vi "Communication - TD PID Data (FGV).vi"(7 "Action":T2=enum."Write", 8 "error in (no error)":errorcluster, 11 "TD PID SV":T1) -> (0 "error out":errorcluster, 3 "TD PID SV out":T1)   [LabVIEW 2019]
uses:
  Controls/FGV States.ctl
  Controls/Communication - TD PID.ctl
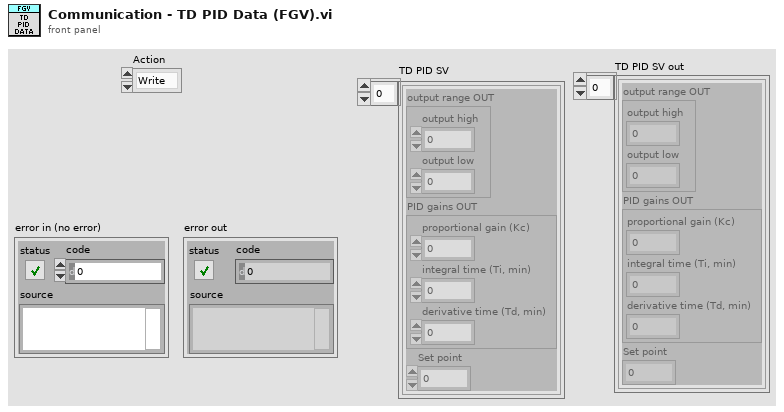
[diagram p1: front panel]
types:
  T1 = typedef "Communication - TD PID.ctl" = cluster{"output range OUT":cluster{"output high":dbl, "output low":dbl}, "PID gains OUT":cluster{"proportional gain (Kc)":dbl, "integral time (Ti, min)":dbl, "derivative time (Td, min)":dbl}, "Set point":dbl}[]
  T2 = typedef "FGV States.ctl" = enum16{"Read", "Write"}
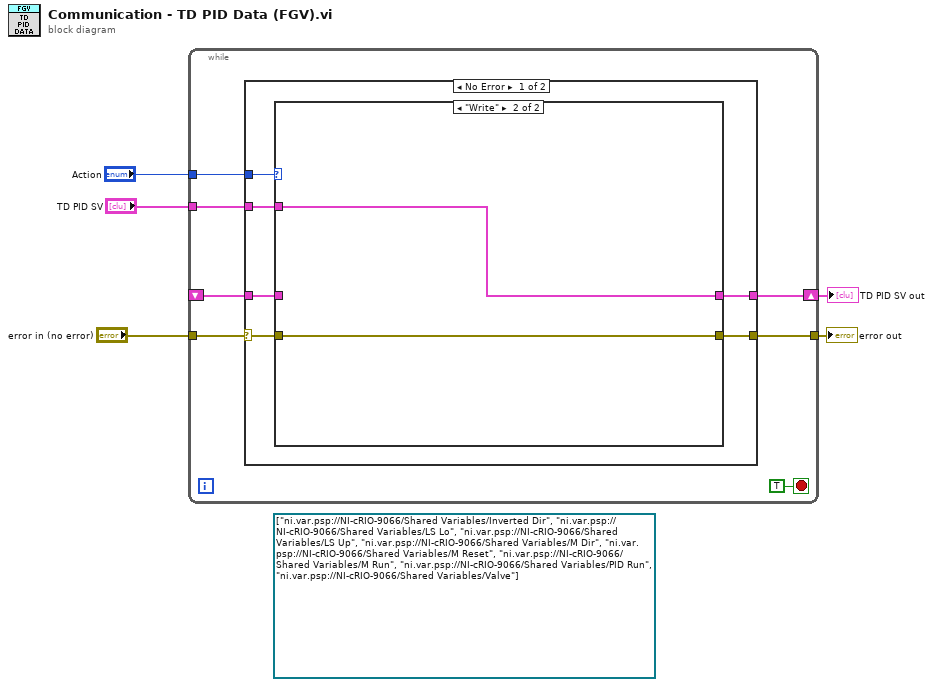
[diagram p0: block diagram]
diagram:
  (unwired) refnum<k21>[] ["ni.var.psp://NI-cRIO-9066/Shared Variables/Inverted Dir", "ni.var.psp://NI-cRIO-9066/Shared Variables/LS Lo", "ni.var.psp://NI-cRIO-9066/Shared Variables/LS Up", "ni.var.psp://NI-cRIO-9066/Shared Variables/M Dir", "ni.var.psp://NI-cRIO-9066/Shared Variables/M Reset", "ni.var.psp://NI-cRIO-9066/Shared Variables/M Run", "ni.var.psp://NI-cRIO-9066/Shared Variables/PID Run", "ni.var.psp://NI-cRIO-9066/Shared Variables/Valve"]
  n1 = while {
    tunnel: "Action" -> [w12]
    tunnel: "TD PID SV" -> [w10]
    shift-right: [w11] -> w1
    shift-left: _ -> [w9]
    tunnel: "error in (no error)" -> [w7]
    tunnel: [w6] -> w3
    stop <- TRUE stop-if-true
    n2 = case shown="No Error" w7 {
      selector: w7 -> [w13 w23]
      tunnel: w12 -> [w18 _]
      tunnel: [w17 w24] -> w11
      tunnel: w10 -> [w16 _]
      tunnel: w9 -> [w15 w24]
      tunnel: [w14 w23] -> w6
      frame No Error {
        n3 = case shown="\"Write\"" w18 {
          tunnel: [w20 w22] -> w17
          tunnel: w16 -> [_ w22]
          tunnel: w15 -> [w20 _]
          tunnel: [w19 w21] -> w14
          tunnel: w13 -> [w19 w21]
          frame "Read", Default {
          }
          frame "Write" {
          }
        }
      }
      frame Error {
      }
    }
  }
  "error out" <- w3
  "TD PID SV out" <- w1
